vi "Create (Structured Append).vi"(7 "Correction Level (Default: Level L)":T1, 8 "error in (no error)":errorcluster, 11 "Number of Structures":u8=2) -> (0 "error out":errorcluster, 3 "QR Code Encoder":refnum<class "QR Code Encoder.lvclass">)   [LabVIEW 2020, in "feature_detection.lvlib" / "QR Code Encoder.lvclass"]
doc: "Create a QR Code Generator."
uses:
  QR Code Encoder.lvclass
  Correction Levels.ctl
  QR Code Encoder.lvclass/QR Code Encoder.ctl
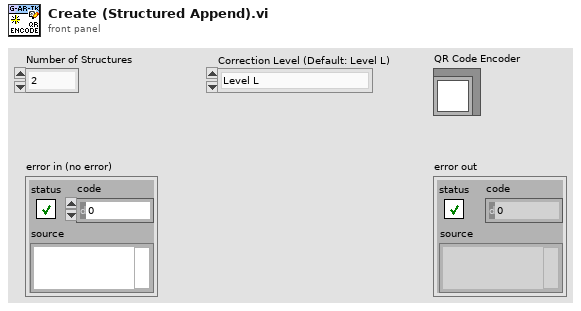
[diagram p1: front panel]
types:
  T1 = typedef "feature_detection.lvlib/QR Code Encoder.lvclass/Correction Levels.ctl" = enum16{"Level L", "Level M", "Level Q", "Level H"}
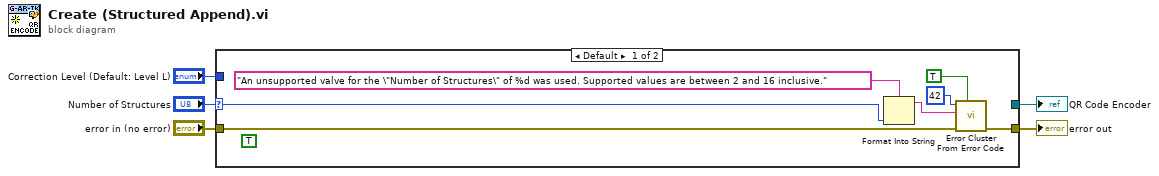
[diagram p0: block diagram]
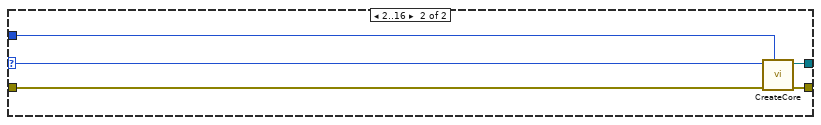
[diagram p2: hidden frame]
diagram:
  n1 = case shown="Default" "Number of Structures" {
    selector: "Number of Structures" -> [w9 w13]
    tunnel: "error in (no error)" -> [w12 w17]
    tunnel: [w11 w16] -> w4
    tunnel: [_ w15] -> w3
    tunnel: "Correction Level (Default: Level L)" -> [_ w14]
    frame Default {
      (unwired) TRUE ("show call chain? (False)")
      n2 = Format Into String(format string="An unsupported valve for the \"Number of Structures\" of %d was used. Supported values are between 2 and 16 inclusive.", w9) -> (resulting string=w8:string)  [unwired: 2 in, 1 out]
      n3 = call <vilib>:"Error Cluster From Error Code.vi"("show call chain? (False)"=TRUE, "error in (no error)"=w12, "error message (\"\")"=w8, "error code (0)"=42) -> ("error out"=w11:errorcluster)  [unwired: 5 in]
    }
    frame 2..16 {
      n4 = call "CreateCore.vi"("Correction Levels"=w14, "error in (no error)"=w17, "n_qr_codes"=w13) -> ("error out"=w16:errorcluster, "QR Code Encoder"=w15:refnum<class "QR Code Encoder.lvclass">)  [unwired: 7 in]
    }
  }
  "error out" <- w4
  "QR Code Encoder" <- w3
